vi "UserVars-Get PDF.vi"(0 "Expr in":string, 11 "error in (no error)":errorcluster) -> (4 "Expr out":string, 6 "X":dbl[][](array[numeric]), 8 "PDF":dbl[][](array[numeric]), 10 "Ref Pts":dbl[][](array[numeric]), 13 "mass function":bool, 14 "Vars":string[](array[string]), 15 "error out":errorcluster)   [LabVIEW 2020]
uses:
  <vilib>/Analysis/1siggen.llb/Ramp Pattern by Samples.vi
  <vilib>/gmath/statdist.llb/Normal PDF.vi
  <vilib>/gmath/statdist.llb/Exp PDF.vi
  <vilib>/gmath/statdist.llb/Uniform PDF.vi
  <vilib>/regexp/Match Regular Expression.xnode
  <vilib>/gmath/NI_Gmath.lvlib
  <vilib>/Analysis/NI_AALBase.lvlib
panel:
  in  "samples":i32=1000
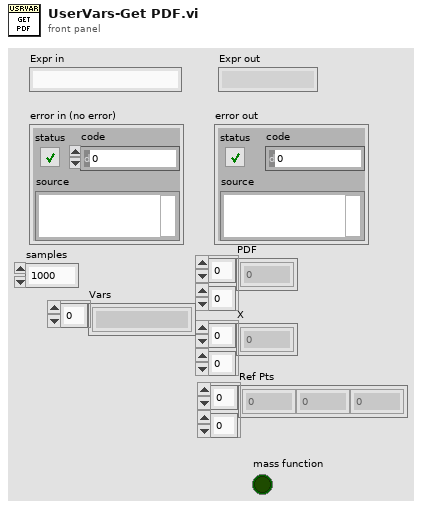
[diagram p1: front panel]
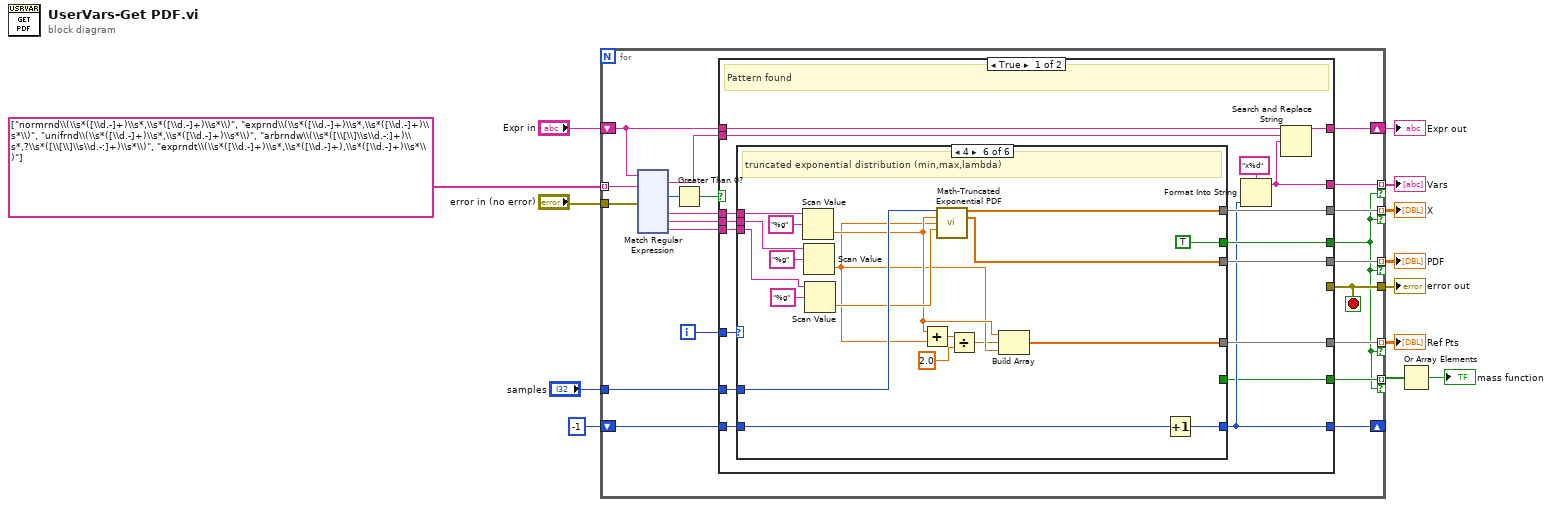
[diagram p0: block diagram]
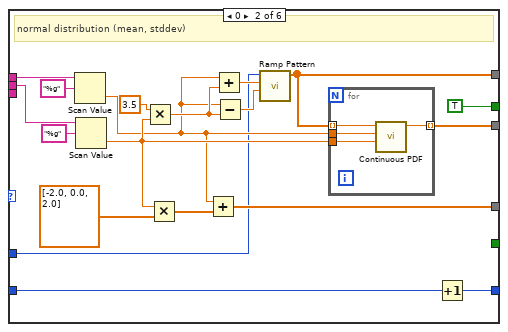
[diagram p3: hidden frame]
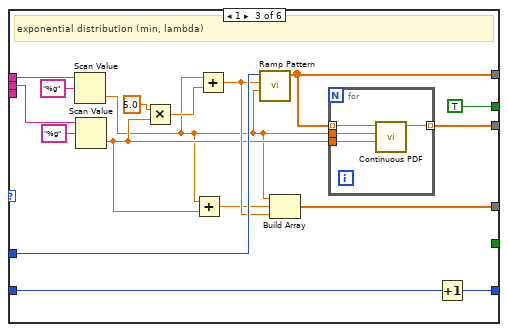
[diagram p4: hidden frame]
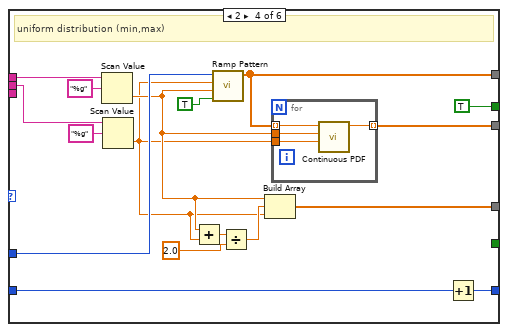
[diagram p5: hidden frame]
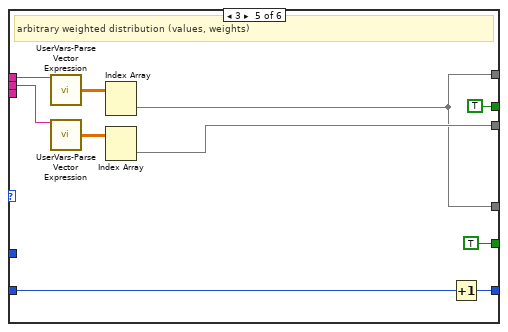
[diagram p6: hidden frame]
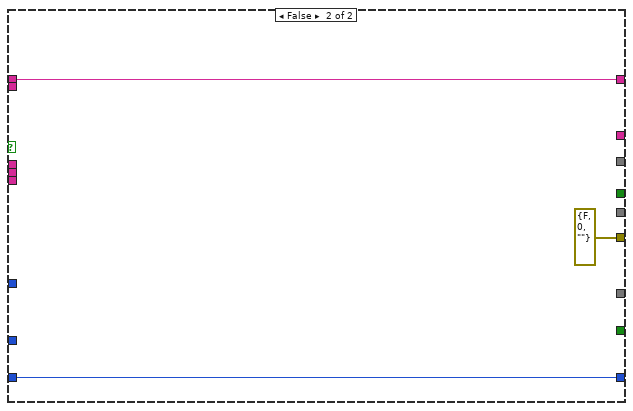
[diagram p7: hidden frame]
diagram:
  n1 = for {
    shift-right: [w31] -> w10
    shift-left: "Expr in" -> [w32]
    tunnel: string[] ["normrnd\\(\\s*([\\d.-]+)\\s*,\\s*([\\d.-]+)\\s*\\)", "exprnd\\(\\s*([\\d.-]+)\\s*,\\s*([\\d.-]+)\\s*\\)", "unifrnd\\(\\s*([\\d.-]+)\\s*,\\s*([\\d.-]+)\\s*\\)", "arbrndw\\(\\s*([\\[\\]\\s\\d.-:]+)\\s*,?\\s*([\\[\\]\\s\\d.-:]+)\\s*\\)", "exprndt\\(\\s*([\\d.-]+)\\s*,\\s*([\\d.-]+),\\s*([\\d.-]+)\\s*\\)"] ("String") -> [w24] mode=indexing
    tunnel: "error in (no error)" -> [w34]
    tunnel: [w15] -> w9
    tunnel: [w23] -> w8 mode=indexing if=w14
    tunnel: [w22] -> w7 mode=indexing if=w14
    tunnel: [w21] -> w6 mode=indexing if=w14
    tunnel: "samples" -> [w20]
    tunnel: [w19] -> w4 mode=indexing if=w14
    shift-right: [w17] -> _
    shift-left: -1 -> [w18]
    tunnel: [w16] -> w2 mode=indexing if=w14
    i -> [w26]
    stop <- w15 stop-if-true
    n2 = xnode "Match Regular Expression"("input string"=w32, "regular expression"=w24, "error in"=w34) -> ("whole match"=w30:string, "offset past match"=w33:i32, "submatch 1"=w29:string, "submatch 2"=w28:string, "submatch 3"=w25:string)  [unwired: 3 in, 3 out]
    n3 = Greater Than 0?(x=w33) -> (x > 0?=w27:bool)
    n4 = case shown="True" w27 {
      tunnel: w32 -> [w47 w149]
      tunnel: [w45 w149] -> w31
      tunnel: w30 -> [w46 _]
      tunnel: w29 -> [w50 _]
      tunnel: w28 -> [w49 _]
      tunnel: w26 -> [w51 _]
      tunnel: w25 -> [w48 _]
      tunnel: [w44 _] -> w23
      tunnel: [w43 _] -> w14
      tunnel: [w42 _] -> w22
      tunnel: [w41 _] -> w21
      tunnel: w20 -> [w40 _]
      tunnel: [w38 _] -> w19
      tunnel: w18 -> [w39 w148]
      tunnel: [w36 w148] -> w17
      tunnel: [w35 _] -> w16
      tunnel: [_ errorcluster {"status"=FALSE, "code"=0, "source"=""} ("error constant")] -> w15
      frame True {
        # "Pattern found"
        n5 = case shown="4" w51 {
          tunnel: w50 -> [_ w71 w92 w113 w127 w146]
          tunnel: w49 -> [_ w68 w89 w110 w124 w138]
          tunnel: w48 -> [_ _ _ _ _ w128]
          tunnel: [_ w63 w86 w107 w120 w129] -> w44
          tunnel: [_ TRUE TRUE TRUE TRUE TRUE] -> w43
          tunnel: [_ w61 w84 w108 w119 w130] -> w42
          tunnel: [_ w56 w80 w106 w119 w140] -> w41
          tunnel: w40 -> [_ w55 w83 w109 _ w137]
          tunnel: w39 -> [w52 w54 w82 w98 w123 w142]
          tunnel: [w52 w53 w81 w97 w122 w141] -> w36
          tunnel: [_ _ _ _ TRUE _] -> w35
          frame -1, Default {
          }
          frame 0 {
            # "normal distribution (mean, stddev)"
            n6 = Scan Value(string=w71, format string="%g") -> (value=w58:dbl)  [unwired: 1 in, 1 out]
            n7 = Scan Value(string=w68, format string="%g") -> (value=w60:dbl)  [unwired: 1 in, 1 out]
            n8 = Multiply(x=3.5 ("y"), y=w60) -> (x*y=w66:dbl)
            n9 = Multiply(x=w60, y=dbl[] [-2.0, 0.0, 2.0]) -> (x*y=w57:dbl[])
            n10 = Add(x=w58, y=w57) -> (x+y=w56:dbl[])
            n11 = Add(x=w58, y=w66) -> (x+y=w65:dbl)
            n12 = Subtract(x=w58, y=w66) -> (x-y=w64:dbl)
            n13 = call-poly <vilib>:"Ramp Pattern.vi"("start"=w64, "end"=w65, "samples"=w55) -> ("Ramp Pattern"=w61:dbl[])  [unwired: 7 in, 1 out]
            n14 = for {
              tunnel: w60 -> [w75]
              tunnel: w58 -> [w74]
              tunnel: w61 -> [w73] mode=indexing
              tunnel: [w72] -> w63 mode=indexing
              n15 = call-poly <vilib>:"Continuous PDF.vi"("std"=w75, "mean"=w74, "x"=w73) -> ("pdf(x)"=w72:dbl)  [unwired: 7 in, 1 out]
            }
            n16 = Increment(x=w54) -> (x+1=w53:i32)
          }
          frame 1 {
            # "exponential distribution (min, lambda)"
            n17 = Scan Value(string=w92, format string="%g") -> (value=w76:dbl)  [unwired: 1 in, 1 out]
            n18 = Scan Value(string=w89, format string="%g") -> (value=w78:dbl)  [unwired: 1 in, 1 out]
            n19 = Multiply(x=5.0 ("y"), y=w78) -> (x*y=w87:dbl)
            n20 = Add(x=w76, y=w78) -> (x+y=w77:dbl)
            n21 = Add(x=w76, y=w87) -> (x+y=w79:dbl)
            n22 = call-poly <vilib>:"Ramp Pattern.vi"("start"=w76, "end"=w79, "samples"=w83) -> ("Ramp Pattern"=w84:dbl[])  [unwired: 7 in, 1 out]
            n23 = Build Array(w76, w77, w79) -> (w80:dbl[])
            n24 = for {
              tunnel: w78 -> [w96]
              tunnel: w76 -> [w95]
              tunnel: w84 -> [w94] mode=indexing
              tunnel: [w93] -> w86 mode=indexing
              n25 = call-poly <vilib>:"Continuous PDF.vi"("b"=w96, "a"=w95, "x"=w94) -> ("pdf(x)"=w93:dbl)  [unwired: 7 in, 1 out]
            }
            n26 = Increment(x=w82) -> (x+1=w81:i32)
          }
          frame 2 {
            # "uniform distribution (min,max)"
            n27 = Scan Value(string=w113, format string="%g") -> (value=w102:dbl)  [unwired: 1 in, 1 out]
            n28 = Scan Value(string=w110, format string="%g") -> (value=w101:dbl)  [unwired: 1 in, 1 out]
            n29 = Add(x=w102, y=w101) -> (x+y=w105:dbl)
            n30 = call-poly <vilib>:"Ramp Pattern.vi"("exclude end?"=TRUE, "start"=w102, "end"=w101, "samples"=w109) -> ("Ramp Pattern"=w108:dbl[])  [unwired: 6 in, 1 out]
            n31 = Divide(x=w105, y=2.0) -> (x/y=w103:dbl)
            n32 = Build Array(w102, w103, w101) -> (w106:dbl[])
            n33 = for {
              tunnel: w101 -> [w117]
              tunnel: w102 -> [w116]
              tunnel: w108 -> [w115] mode=indexing
              tunnel: [w114] -> w107 mode=indexing
              n34 = call-poly <vilib>:"Continuous PDF.vi"("xmax"=w117, "xmin"=w116, "x"=w115) -> ("pdf(x)"=w114:dbl)  [unwired: 7 in, 1 out]
            }
            n35 = Increment(x=w98) -> (x+1=w97:i32)
          }
          frame 3 {
            # "arbitrary weighted distribution (values, weights)"
            n36 = call "UserVars-Parse Vector Expression.vi"("Expression In"=w127) -> ("values"=w126:dbl[][])  [unwired: 11 in, 3 out]
            n37 = call "UserVars-Parse Vector Expression.vi"("Expression In"=w124) -> ("values"=w125:dbl[][])  [unwired: 11 in, 3 out]
            n38 = Index Array(array=w126) -> (element=w119:dbl[])  [unwired: 2 in]
            n39 = Index Array(array=w125) -> (element=w120:dbl[])  [unwired: 2 in]
            n40 = Increment(x=w123) -> (x+1=w122:i32)
          }
          frame 4 {
            # "truncated exponential distribution (min,max,lambda)"
            n41 = Scan Value(string=w146, format string="%g") -> (value=w135:dbl)  [unwired: 1 in, 1 out]
            n42 = Scan Value(string=w138, format string="%g") -> (value=w134:dbl)  [unwired: 1 in, 1 out]
            n43 = Scan Value(string=w128, format string="%g") -> (value=w136:dbl)  [unwired: 1 in, 1 out]
            n44 = Add(x=w135, y=w134) -> (x+y=w133:dbl)
            n45 = call "Math-Truncated Exponential PDF.vi"("samples"=w137, "Min"=w135, "Max"=w134, "Lambda"=w136) -> ("X"=w130:dbl[], "PDF(X)"=w129:dbl[])  [unwired: 10 in]
            n46 = Divide(x=w133, y=2.0) -> (x/y=w131:dbl)
            n47 = Build Array(w135, w131, w134) -> (w140:dbl[])
            n48 = Increment(x=w142) -> (x+1=w141:i32)
          }
        }
        n49 = Format Into String(format string="x%d", w36) -> (resulting string=w38:string)  [unwired: 2 in, 1 out]
        n50 = Search and Replace String(input string=w47, search string=w46, replace string=w38) -> (result string=w45:string)  [unwired: 5 in, 3 out]
      }
      frame False {
      }
    }
  }
  "error out" <- w9
  "Expr out" <- w10
  "PDF" <- w8
  "X" <- w7
  "Ref Pts" <- w6
  "Vars" <- w4
  n51 = Or Array Elements(Boolean array=w2) -> (logical OR=→"mass function":bool)
